vi "update.vi"(8 "error in (no error)":errorcluster, 11 "HSDIO in":refnum<class "HSDIO.lvclass">) -> (0 "error out":errorcluster, 3 "HSDIO out":refnum<class "HSDIO.lvclass">)   [LabVIEW 2013, in "HSDIO.lvclass"]
uses:
  HSDIO.lvclass
  HSDIO.lvclass/HSDIO.ctl
  Globals.vi
  <instrlib>/niHSDIO/niHSDIO.llb/niHSDIO Write Named Waveform (WDT).vi
panel:
  out "transitions":u32[](array[numeric])
  out "states":u8[][](array[numeric])
  out "output waveform":digitaldata
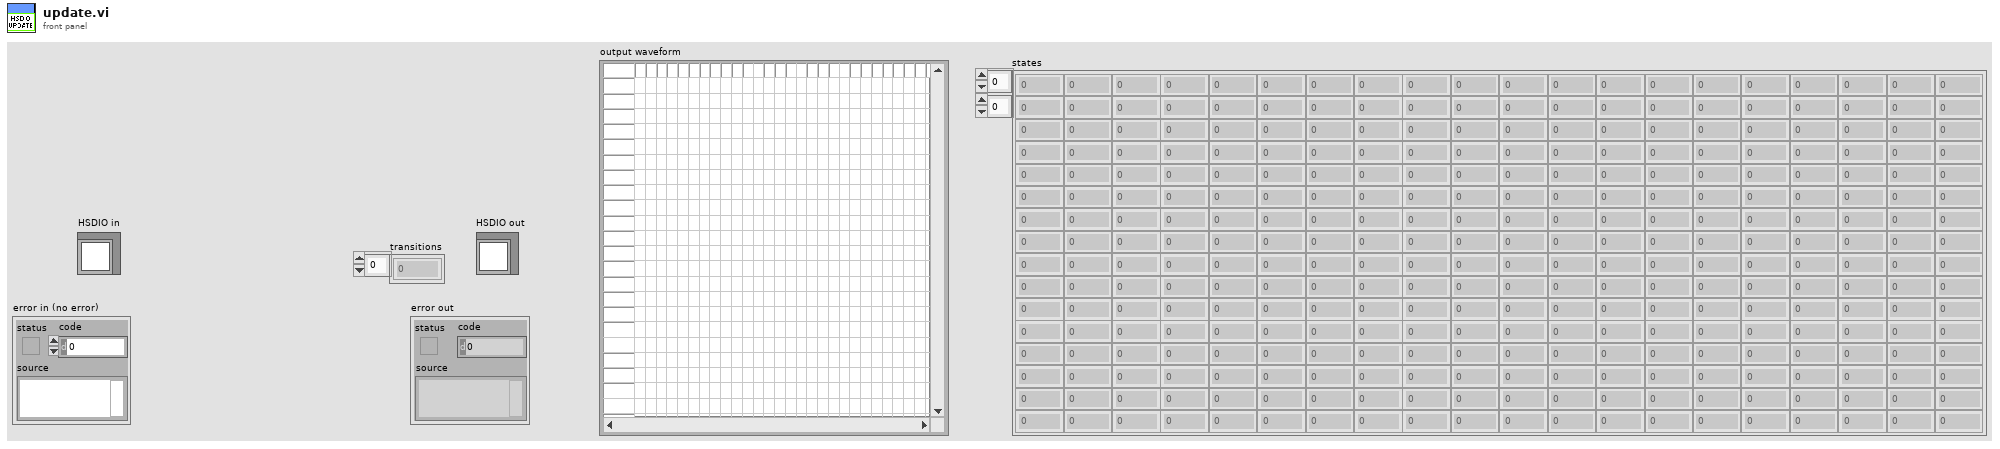
[diagram p1: front panel]
types:
  T1 = typedef "HSDIO.lvclass/waveform.ctl" = cluster{"name":string, "transitions":u32[], "states":u8[][]}
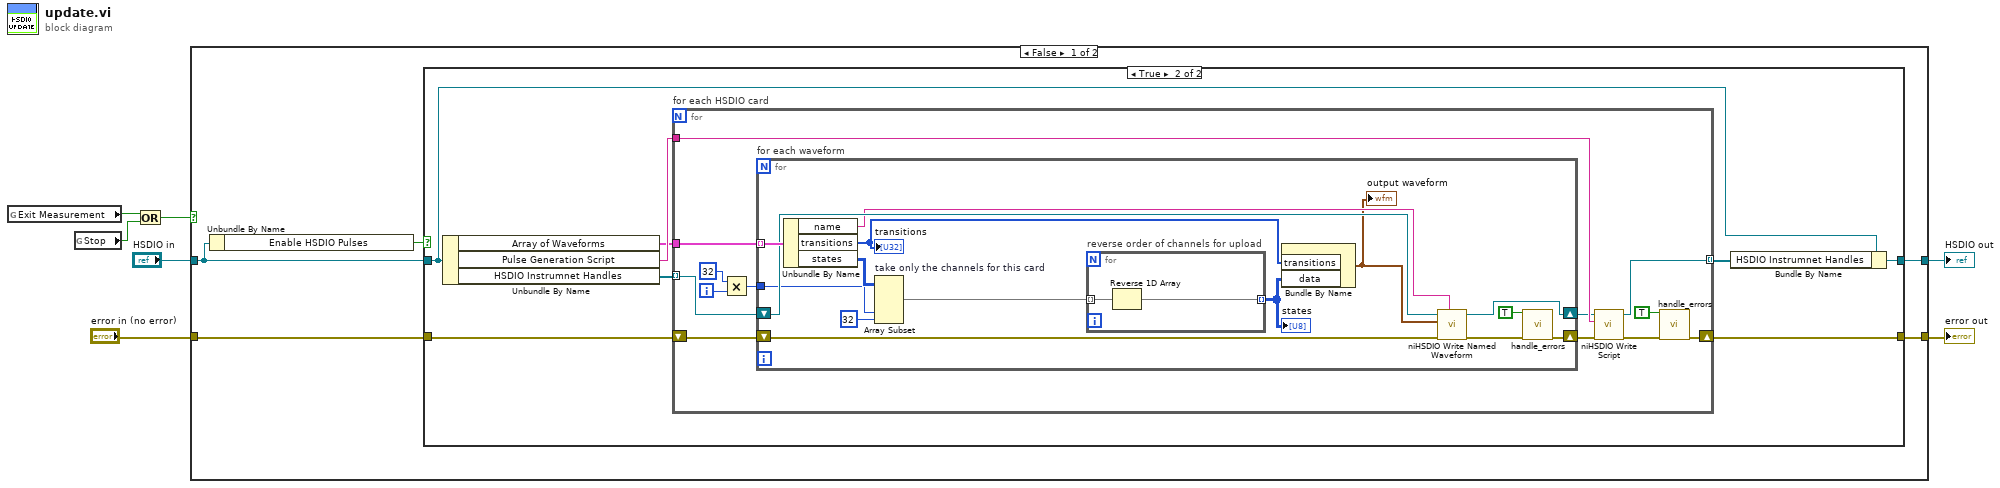
[diagram p0: block diagram]
diagram:
  n1 = global read "Globals.vi" "Exit Measurement"() -> (w3:bool)
  n2 = global read "Globals.vi" "Stop"() -> (w2:bool)
  n3 = Or(x=w3, y=w2) -> (x .or. y?=w1:bool)
  n4 = case shown="False" w1 {
    tunnel: [w8 w53] -> w5
    tunnel: [w10 w54] -> w6
    tunnel: "HSDIO in" -> [w11 w54]
    tunnel: "error in (no error)" -> [w9 w53]
    frame False {
      n5 = Unbundle By Name(w11) -> ("Enable HSDIO Pulses"=w12:bool)
      n6 = case shown="True" w12 {
        tunnel: w11 -> [w14 w20]
        tunnel: [w14 w21] -> w10
        tunnel: w9 -> [w13 w17]
        tunnel: [w13 w16] -> w8
        frame False {
        }
        frame True {
          n7 = Unbundle By Name(w20) -> ("Array of Waveforms"=w15:T1[], "Pulse Generation Script"=w19:string, "HSDIO Instrumnet Handles"=w18:refnum<k15>[])
          n8 = for "for each HSDIO card" {
            tunnel: [w35] -> w22 mode=indexing
            tunnel: w19 -> [w34]
            tunnel: w18 -> [w33] mode=indexing
            tunnel: w15 -> [w28]
            shift-right: [w29] -> w16
            shift-left: w17 -> [w30]
            i -> [w25]
            n9 = Multiply(x=32 ("length"), y=w25) -> (x*y=w23:i32)
            n10 = for "for each waveform" {
              tunnel: w28 -> [w50] mode=indexing
              shift-right: [w45] -> w31
              shift-left: w30 -> [w46]
              shift-right: [w47] -> w32
              shift-left: w33 -> [w48]
              tunnel: w23 -> [w36]
              n11 = Unbundle By Name(w50) -> ("name"=w44:string, "transitions"=w49:u32[], "states"=w41:u8[][])
              "transitions" <- w49
              n12 = Array Subset "take only the channels for this card"(array=w41, index (col)=w36, length (col)=32 ("length")) -> (w38:u8[][])  [unwired: 2 in]
              n13 = for "reverse order of channels for upload" {
                tunnel: w38 -> [w52] mode=indexing
                tunnel: [w51] -> w42 mode=indexing
                n14 = Reverse 1D Array(array=w52) -> (reversed array=w51:u8[])
              }
              "states" <- w42
              n15 = Bundle By Name("transitions"=w49, "data"=w42) -> (w43:digitaldata)  [unwired: 1 in]
              "output waveform" <- w43
              n16 = call-poly <instrlib>:"niHSDIO Write Named Waveform.vi"("waveform name (default:\"\")"=w44, "error in (no error)"=w46, "data"=w43, "instrument handle"=w48) -> ("error out"=w40:errorcluster, "instrument handle out"=w47:refnum<k15>)  [unwired: 6 in]
              n17 = call "handle_errors.vi"("Exit Operation"=TRUE ("Exit Measurement"), "error in (no error)"=w40) -> ("error out"=w45:errorcluster)  [unwired: 13 in]
            }
            n18 = call <instrlib>:"niHSDIO Write Script.vi"("error in (no error)"=w31, "script"=w34, "instrument handle"=w32) -> ("error out"=w27:errorcluster, "instrument handle out"=w35:refnum<k15>)  [unwired: 7 in]
            n19 = call "handle_errors.vi"("Exit Operation"=TRUE ("Exit Measurement"), "error in (no error)"=w27) -> ("error out"=w29:errorcluster)  [unwired: 13 in]
          }
          n20 = Bundle By Name(cluster=w20, "HSDIO Instrumnet Handles"=w22) -> (w21:refnum<class "HSDIO.lvclass">)
        }
      }
    }
    frame True {
    }
  }
  "error out" <- w5
  "HSDIO out" <- w6
